vi "Logging Read One.vi"(4 "error in (no error)":errorcluster, 7 "LoggingDevRef":T5) -> (0 "error out":errorcluster, 1 "EOF":bool, 2 "Output":T1, 3 "LoggingDevRef":T5)   [LabVIEW 2012, in "femtoRoboLib.lvlib"]
uses:
  femtoRoboLib.lvlib
  LoggingDevRef.ctl
  Log Entry Block.ctl
  Log Entry.ctl
  Log Value Type.ctl
  Log Value Cluster.ctl
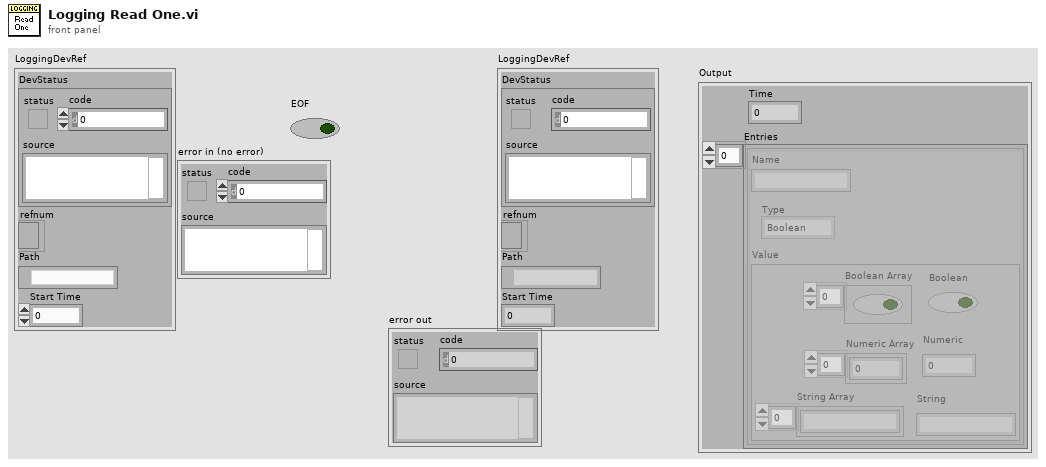
[diagram p1: front panel]
types:
  T1 = typedef "femtoRoboLib.lvlib/Log Entry Block.ctl" = cluster{"Entries":T2[], "Time":u32}
  T2 = typedef "femtoRoboLib.lvlib/Log Entry.ctl" = cluster{"Name":string, "Type":T3, "Value":T4}
  T3 = typedef "femtoRoboLib.lvlib/Log Value Type.ctl" = enum16{"Boolean", "Numeric", "String", "Boolean Array", "Numeric Array", "String Array"}
  T4 = typedef "femtoRoboLib.lvlib/Log Value Cluster.ctl" = cluster{"Boolean Array":bool[], "Boolean":bool, "Numeric Array":dbl[], "Numeric":dbl, "String Array":string[], "String":string}
  T5 = typedef "femtoRoboLib.lvlib/LoggingDevRef.ctl" = cluster{"DevStatus":errorcluster, "refnum":refnum<file>, "Path":path, "Start Time":u32}
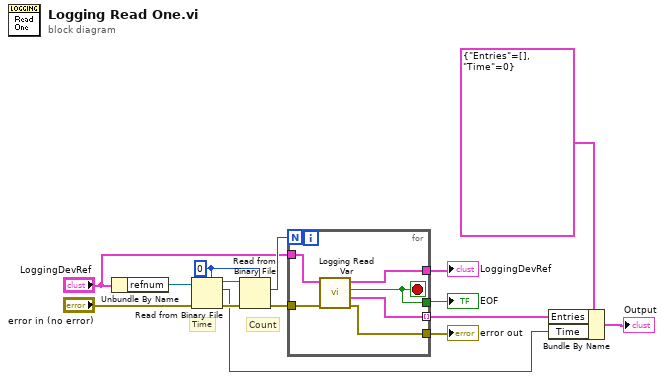
[diagram p0: block diagram]
diagram:
  w14 = u32 0
  # "Count"
  # "Time"
  n1 = Unbundle By Name("LoggingDevRef") -> ("refnum"=w2:refnum<file>)
  n2 = Read from Binary File(5:w14, 8:"error in (no error)", 11:w2) -> (0:w11:errorcluster, 2:w3:u32, 3:w15:refnum<file>)  [unwired: 3 in, 1 out]
  n3 = Read from Binary File(5:w14, 8:w11, 11:w15) -> (0:w10:errorcluster, 2:w13:u32)  [unwired: 3 in, 2 out]
  n4 = for {
    N: w13 -> [_]
    tunnel: "LoggingDevRef" -> [w19]
    tunnel: w10 -> [w21]
    tunnel: [w20] -> w9
    tunnel: [w18] -> w8
    tunnel: [w17] -> w4 mode=indexing
    tunnel: [w16] -> w7
    stop <- w16 stop-if-true
    n5 = call "Logging Read Var.vi"("error in (no error)"=w21, "LoggingDevRef"=w19) -> ("error out"=w20:errorcluster, "Output"=w17:T2, "EOF"=w16:bool, "LoggingDevRef"=w18:T5)  [unwired: 2 in]
  }
  "EOF" <- w7
  "LoggingDevRef" <- w8
  "error out" <- w9
  n6 = Bundle By Name(cluster=T1 {"Entries"=[], "Time"=0} ("Output"), "Entries"=w4, "Time"=w3) -> (→"Output":T1)
